vi "FT_Error_codes.vi"() -> ()   [LabVIEW 2019]
panel:
  in  "STATUS_CODES":string[](array[string])=["OK", "INVALID HANDLE", "DEVICE NOT FOUND", "DEVICE NOT OPENED", "IO ERROR", "INSUFFICIENT RESOURCES", "INVALID PARAMETER", "INVALID BAUD RATE", "DEVICE NOT OPENED FOR ERASE", "DEVICE NOT OPENED FOR WRITE", "FAILED TO WRITE DEVICE", "EEPROM READ FAILED", "EEPROM WRITE FAILED", "EEPROM ERASE FAILED", "EEPROM NOT PRESENT", "EEPROM NOT PROGRAMMED", "INVALID ARGS", "NOT SUPPORTED", "OTHER ERROR"]
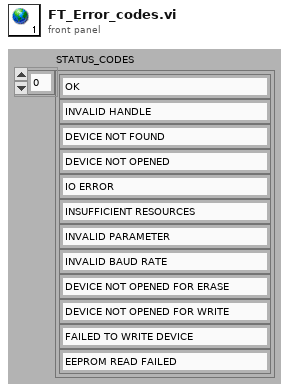
[diagram p1: front panel]
diagram:
